vi "Barcode 2D_Main Function.vi"(8 "error in (no error)":errorcluster, 10 "2D Barcode Parameter in":T1={"ROI"={"Global Rectangle"=[], "Contours"=[]}, "Barcode Type"=enum."PDF417", "Data Matrix Parameter"={"Data Matrix Description Options"={"Aspect Ratio"=0.0, "Rows"=0, "Columns"=0, "Rectangle"=FALSE, "ECC"=-2, "Barcode Polarity"=0, "Cell Fill Percentage"=-2, "Minimum Border Integrity %"=80.0, "Mirror Mode"=-2}, "Data Matrix Search Options"={"Rotation Mode"=enum."Unlimited", "Skip Location?"=FALSE, "Edge Threshold"=30, "Demodulation Mode"=-2, "Cell Sample Size"=-2, "Cell Filter Mode"=-2, "Skew Degrees Allowed"=5, "Maximum Iterations"=500, "Initial Search Vector Width"=5}, "Data Matrix Size Options"={"Data Matrix Size"={"Minimum Size"=0, "Maximum Size"=0}, "Quiet Zone Width"=10}, "Advanced Options"=[]}, "PDF147 Search Mode"=enum."Multiple Barcodes", "QR Code Parameter"={"QR Search Options"={"Rotation Mode"=enum."Unlimited", "Skip Location?"=FALSE, "Edge Threshold"=30, "Demodulation Mode"=-2, "Cell Sample Size"=-2, "Cell Filter Mode"=-2, "Skew Degrees Allowed"=5}, "QR Description Options"={"Matrix Size (cells)"=0, "Barcode Polarity"=-2, "Mirror Mode"=-2, "QR Model"=0}, "QR Code Cell Size (pixels)"={"Minimum Size"=3, "Maximum Size"=7}}} {"QR Code Parameter"."QR Description Options"."Mirror Mode" items=["Auto-detect"=-2, "Normal"=0, "Mirrored"=1]; "QR Code Parameter"."QR Description Options"."Matrix Size (cells)" items=["Auto-detect"=0, "11x11 - Version 1 (Micro QR Only)"=11, "13x13 - Version 2 (Micro QR Only)"=13, "15x15 - Version 3 (Micro QR Only)"=15, "17x17 - Version 4 (Micro QR Only)"=17, "21x21 - Version 1"=21, "25x25 - Version 2"=25, "29x29 - Version 3"=29, "33x33 - Version 4"=33, "37x37 - Version 5"=37, "41x41 - Version 6"=41, "45x45 - Version 7"=45, "49x49 - Version 8"=49, "53x53 - Version 9"=53, "57x57 - Version 10"=57, "61x61 - Version 11"=61, "65x65 - Version 12"=65, "69x69 - Version 13"=69, "73x73 - Version 14"=73, "77x77 - Version 15"=77, "81x81 - Version 16"=81, "85x85 - Version 17"=85, "89x89 - Version 18"=89, "93x93 - Version 19"=93, "97x97 - Version 20"=97, "101x101 - Version 21"=101, "105x105 - Version 22"=105, "109x109 - Version 23"=109, "113x113 - Version 24"=113, "117x117 - Version 25"=117, "121x121 - Version 26"=121, "125x125 - Version 27"=125, "129x129 - Version 28"=129, "133x133 - Version 29"=133, "137x137 - Version 30"=137, "141x141 - Version 31"=141, "145x145 - Version 32"=145, "149x149 - Version 33"=149, "153x153 - Version 34"=153, "157x157 - Version 35"=157, "161x161 - Version 36"=161, "165x165 - Version 37"=165, "169x169 -  Version 38"=169, "173x173 - Version 39"=173, "177x177 - Version 40"=177]; "QR Code Parameter"."QR Description Options"."QR Model" items=["Auto-detect", "Micro", "Model 1", "Model 2"]; "QR Code Parameter"."QR Description Options"."Barcode Polarity" items=["Auto-detect"=-2, "Black on White"=0, "White on Black"=1]; "QR Code Parameter"."QR Search Options"."Cell Filter Mode" items=["Auto-detect"=-2, "Average"=0, "Median"=1, "Central Average"=2, "High Average"=3, "Low Average"=4, "Very High Average"=5, "Very Low Average"=6, "All Filters"=8]; "QR Code Parameter"."QR Search Options"."Cell Sample Size" items=["Auto-detect"=-2, "1x1"=1, "2x2"=2, "3x3"=3, "4x4"=4, "5x5"=5, "6x6"=6, "7x7"=7]; "QR Code Parameter"."QR Search Options"."Demodulation Mode" items=["Auto-detect"=-2, "Histogram"=0, "Local Contrast"=1, "Combination"=2, "All"=3]; "Data Matrix Parameter"."Advanced Options"."Value" format="%.2f"; "Data Matrix Parameter"."Data Matrix Search Options"."Cell Filter Mode" items=["Auto-detect"=-2, "Average"=0, "Median"=1, "Central Average"=2, "High Average"=3, "Low Average"=4, "Very High Average"=5, "Very Low Average"=6, "All Filters"=8]; "Data Matrix Parameter"."Data Matrix Search Options"."Cell Sample Size" items=["Auto-detect"=-2, "1x1"=1, "2x2"=2, "3x3"=3, "4x4"=4, "5x5"=5, "6x6"=6, "7x7"=7]; "Data Matrix Parameter"."Data Matrix Search Options"."Demodulation Mode" items=["Auto-detect"=-2, "Histogram"=0, "Local Contrast"=1, "Combination"=2, "All"=3]; "Data Matrix Parameter"."Data Matrix Description Options"."Mirror Mode" items=["Auto-detect"=-2, "Normal"=0, "Mirrored"=1]; "Data Matrix Parameter"."Data Matrix Description Options"."ECC" items=["Auto-detect"=-2, "ECC 000"=0, "ECC 050"=50, "ECC 080"=80, "ECC 100"=100, "ECC 140"=140, "ECC 000-140"=190, "ECC 200"=200]; "Data Matrix Parameter"."Data Matrix Description Options"."Minimum Border Integrity %" format="%.2f"; "Data Matrix Parameter"."Data Matrix Description Options"."Aspect Ratio" format="%.2f"; "Data Matrix Parameter"."Data Matrix Description Options"."Cell Fill Percentage" items=["Auto-detect"=-2, "< 30%"=0, ">= 30%"=1]; "Data Matrix Parameter"."Data Matrix Description Options"."Barcode Polarity" items=["Auto-detect"=-2, "Black on White"=0, "White on Black"=1]}, 11 "Image In":T17) -> (0 "error out":errorcluster, 1 "Bounding Box":cluster{"x":sgl, "y":sgl}[](array[cluster]), 2 "Data":string, 3 "Image Out":T17)   [LabVIEW 2019]
uses:
  <vilib>/vision/Image Controls.llb/IMAQ Image.ctl
  Controls/Barcode 2D/Analysis_Barcode 2D_Parameter.ctl
  <vilib>/vision/Instrument.llb/Data Matrix Description Options.ctl
  <vilib>/vision/Instrument.llb/ECC Type.ctl
  <vilib>/vision/Instrument.llb/Data Matrix Polarity.ctl
  <vilib>/vision/Instrument.llb/Cell Fill Percentage.ctl
  <vilib>/vision/Instrument.llb/Data Matrix Mirror.ctl
  <vilib>/vision/Instrument.llb/Data Matrix Search Options.ctl
  <vilib>/vision/Instrument.llb/Demodulation Mode.ctl
  <vilib>/vision/Instrument.llb/Cell Sample Size.ctl
  <vilib>/vision/Instrument.llb/Cell Filter Mode.ctl
  <vilib>/vision/Instrument.llb/Data Matrix Size Options.ctl
  <vilib>/vision/Instrument.llb/Data Matrix Advanced Options.ctl
  <vilib>/vision/Instrument.llb/QR Code Search Options.ctl
  <vilib>/vision/Instrument.llb/QR Code Description Options.ctl
  <vilib>/vision/Instrument.llb/QR Code Model Type.ctl
  <vilib>/vision/NI_Vision_Development_Module.lvlib
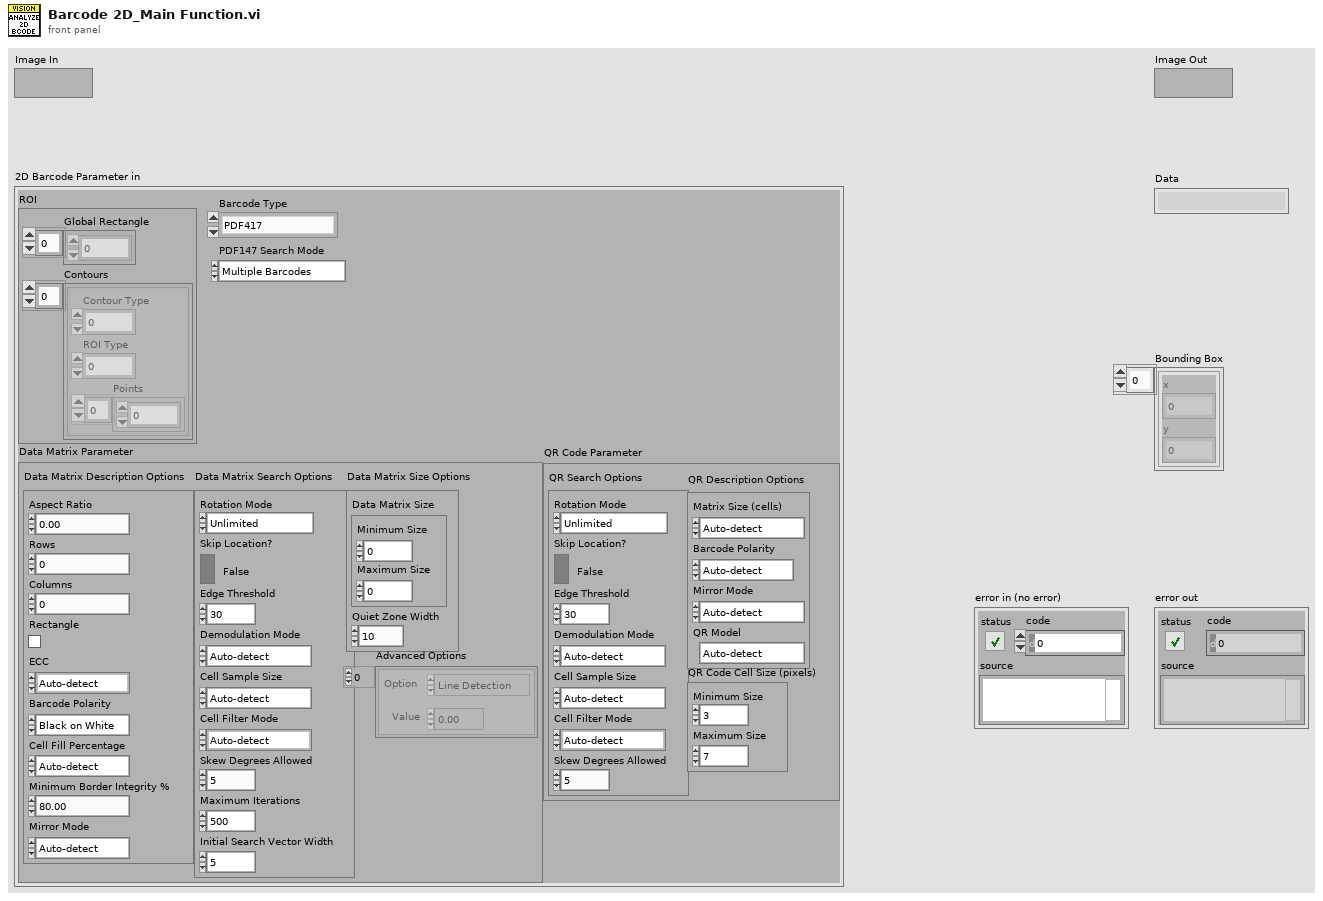
[diagram p1: front panel]
types:
  T1 = typedef "Analysis_Barcode 2D_Parameter.ctl" = cluster{"ROI":cluster{"Global Rectangle":i32[], "Contours":cluster{"Contour Type":u32, "ROI Type":u32, "Points":i32[]}[]}, "Barcode Type":enum16{"Data Matrix", "PDF417", "QR Code"}, "Data Matrix Parameter":cluster{"Data Matrix Description Options":T2, "Data Matrix Search Options":T7, "Data Matrix Size Options":T11, "Advanced Options":T12[]}, "PDF147 Search Mode":T13, "QR Code Parameter":cluster{"QR Search Options":T14, "QR Description Options":T15, "QR Code Cell Size (pixels)":cluster{"Minimum Size":u32, "Maximum Size":u32}}}
  T2 = typedef "Data Matrix Description Options.ctl" = cluster{"Aspect Ratio":sgl, "Rows":u32, "Columns":u32, "Rectangle":bool, "ECC":T3, "Barcode Polarity":T4, "Cell Fill Percentage":T5, "Minimum Border Integrity %":sgl, "Mirror Mode":T6}
  T3 = typedef "ECC Type.ctl" = i32
  T4 = typedef "Data Matrix Polarity.ctl" = i32
  T5 = typedef "Cell Fill Percentage.ctl" = i32
  T6 = typedef "Data Matrix Mirror.ctl" = i32
  T7 = typedef "Data Matrix Search Options.ctl" = cluster{"Rotation Mode":enum32{"Unlimited", "0 Degrees", "90 Degrees", "180 Degrees", "270 Degrees"}, "Skip Location?":bool, "Edge Threshold":u32, "Demodulation Mode":T8, "Cell Sample Size":T9, "Cell Filter Mode":T10, "Skew Degrees Allowed":u32, "Maximum Iterations":u32, "Initial Search Vector Width":u32}
  T8 = typedef "Demodulation Mode.ctl" = i32
  T9 = typedef "Cell Sample Size.ctl" = i32
  T10 = typedef "Cell Filter Mode.ctl" = i32
  T11 = typedef "Data Matrix Size Options.ctl" = cluster{"Data Matrix Size":cluster{"Minimum Size":u32, "Maximum Size":u32}, "Quiet Zone Width":u32}
  T12 = typedef "Data Matrix Advanced Options.ctl" = cluster{"Option":enum32{"Line Detection", "HighLight Filter", "Aggressive", "FNC1", "Refine Bounding Box"}, " Value":dbl}
  T13 = typedef "PDF417 Search Mode" = enum32{"Multiple Barcodes", "Single Barcode, Conservative"}
  T14 = typedef "QR Code Search Options.ctl" = cluster{"Rotation Mode":enum32{"Unlimited", "0 Degrees", "90 Degrees", "180 Degrees", "270 Degrees"}, "Skip Location?":bool, "Edge Threshold":u32, "Demodulation Mode":T8, "Cell Sample Size":T9, "Cell Filter Mode":T10, "Skew Degrees Allowed":u32}
  T15 = typedef "QR Code Description Options.ctl" = cluster{"Matrix Size (cells)":i32, "Barcode Polarity":T4, "Mirror Mode":i32, "QR Model":T16}
  T16 = typedef "QR Code Model Type.ctl" = i32
  T17 = typedef "IMAQ Image.ctl" = refnum<image>
  T18 = cluster{"Global Rectangle":i32[], "Contours":cluster{"Contour Type":u32, "ROI Type":u32, "Points":i32[]}[]}
  T19 = typedef "Data Matrix Report.ctl" = cluster{"Found?":bool, "Binary?":bool, "Data":string, "Bounding Box":cluster{"x":sgl, "y":sgl}[], "Errors Corrected":u32, "Erasures Corrected":u32, "Aspect Ratio":sgl, "Rows":u32, "Columns":u32, "ECC":T3, "Barcode Polarity":T4, "Cell Fill Percentage":T5, "Border Integrity":sgl, "Mirrored?":bool, "Minimum Edge Strength":u32, "Demodulation Mode":T8, "Cell Sample Size":T9, "Cell Filter Mode":T10, "Iterations":u32}
  T20 = typedef "Barcode Report" = cluster{"Type":enum32{"PDF417", "Data Matrix ECC 000", "Data Matrix ECC 050", "Data Matrix ECC 080", "Data Matrix ECC 100", "Data Matrix ECC 140", "Data Matrix ECC 200"}, "Binary":bool, "Data":string, "Bounding Box":cluster{"x":sgl, "y":sgl}[], "Errors Corrected":u32, "Erasures Corrected":u32, "Rows":u32, "Columns":u32}
  T21 = typedef "QR Code Report.ctl" = cluster{"Found?":bool, "Data":string, "Bounding Box":cluster{"x":sgl, "y":sgl}[], "Errors Corrected":u32, "Dimensions (Rows/Cols)":u32, "Version":u32, "QR Model":T16, "Stream Mode":T22, "Barcode Polarity":T4, "Mirrored?":bool, "Append Stream Position":u32, "Size of Append Stream":u32, "First EAN-128 ID":i32, "First Alternate Language ID":i32, "Append Stream ID":u32, "Minimum Edge Strength":u32, "Demodulation Mode":T8, "Cell Sample Size":T9, "Cell Filter Mode":T10}
  T22 = typedef "QR Code Stream Mode Type.ctl" = i32
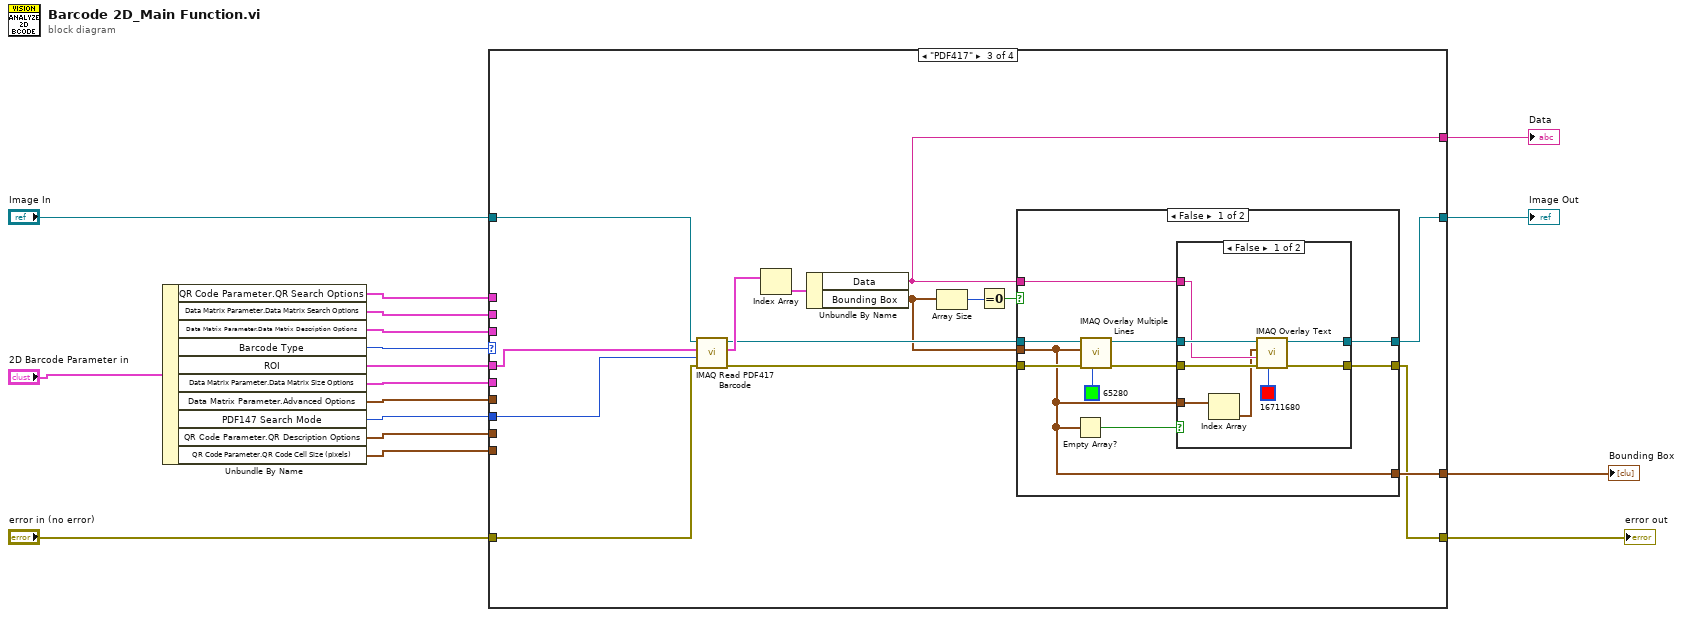
[diagram p0: block diagram]
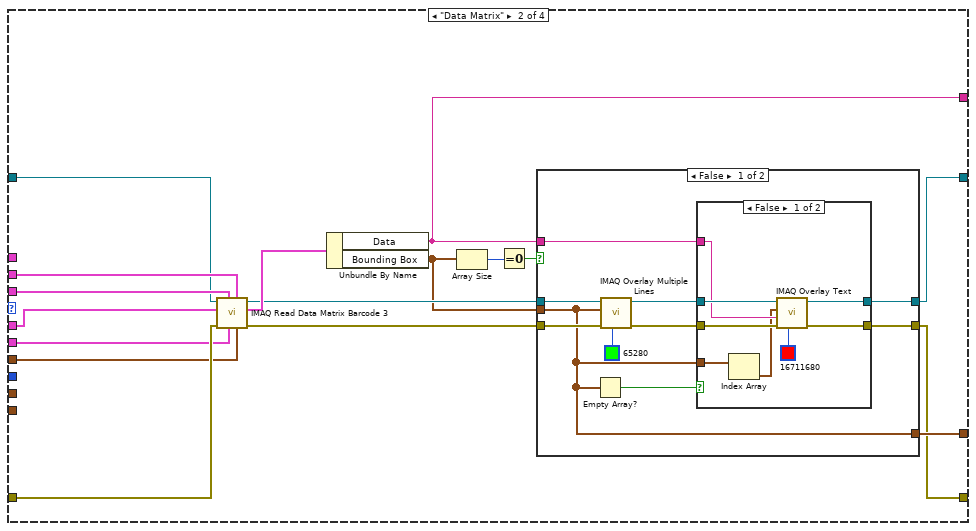
[diagram p3: hidden frame]
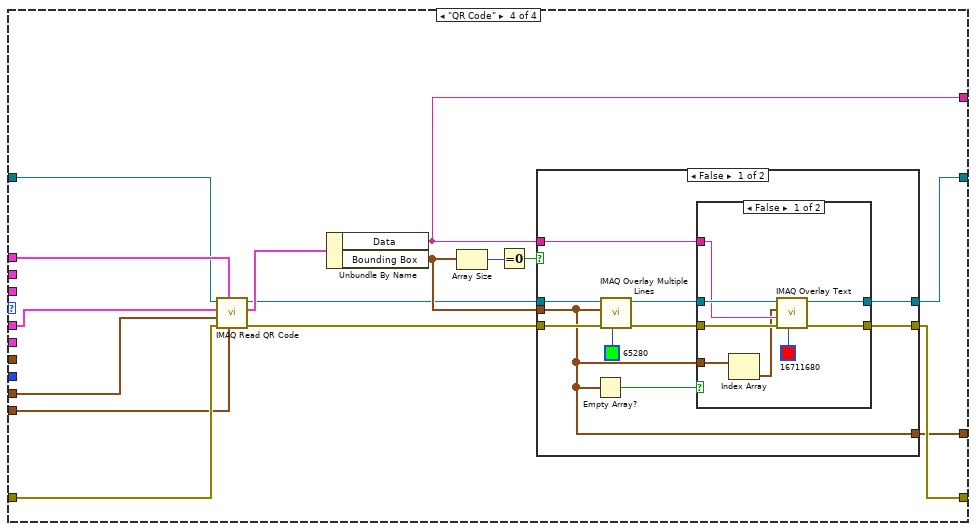
[diagram p8: hidden frame]
diagram:
  n1 = Unbundle By Name("2D Barcode Parameter in") -> ("QR Code Parameter.QR Search Options"=w9:T14, "Data Matrix Parameter.Data Matrix Search Options"=w11:T7, "Data Matrix Parameter.Data Matrix Description Options"=w12:T2, "Barcode Type"=w10:enum16{"Data Matrix", "PDF417", "QR Code"}, "ROI"=w8:T18, "Data Matrix Parameter.Data Matrix Size Options"=w7:T11, "Data Matrix Parameter.Advanced Options"=w6:T12[], "PDF147 Search Mode"=w3:T13, "QR Code Parameter.QR Description Options"=w4:T15, "QR Code Parameter.QR Code Cell Size (pixels)"=w5:cluster{"Minimum Size":u32, "Maximum Size":u32})
  n2 = case shown="\"PDF417\"" w10 {
    tunnel: [w18 w25 w60 w107] -> w1
    tunnel: [w19 w27 w59 w106] -> w17
    tunnel: "error in (no error)" -> [w18 w35 w70 w105]
    tunnel: "Image In" -> [w19 w31 w68 w98]
    tunnel: [_ w26 w61 w102] -> w15
    tunnel: [_ w20 w62 w101] -> w14
    tunnel: w12 -> [_ w33 _ _]
    tunnel: w11 -> [_ w32 _ _]
    tunnel: w9 -> [_ _ _ w100]
    tunnel: w8 -> [_ w30 w69 w99]
    tunnel: w7 -> [_ w29 _ _]
    tunnel: w6 -> [_ w28 _ _]
    tunnel: w4 -> [_ _ _ w96]
    tunnel: w5 -> [_ _ _ w97]
    tunnel: w3 -> [_ _ w67 _]
    frame Default {
    }
    frame "Data Matrix" {
      n3 = call "IMAQ Read Data Matrix Barcode 3"("Advanced Options"=w28, "Data Matrix Search Options"=w32, "Data Matrix Size Options"=w29, "Data Matrix Description Options"=w33, "error in (no error)"=w35, "ROI Descriptor"=w30, "Image"=w31) -> ("error out"=w24:errorcluster, "Data Matrix Report"=w36:T19, "Image (duplicate)"=w23:T17)  [unwired: 1 in, 1 out]
      n4 = Unbundle By Name(w36) -> ("Data"=w20:string, "Bounding Box"=w22:cluster{"x":sgl, "y":sgl}[])
      n5 = Array Size(array=w22) -> (size(s)=w34:i32)
      n6 = Equal To 0?(x=w34) -> (x = 0?=w21:bool)
      n7 = case shown="False" w21 {
        tunnel: w23 -> [w45 w58]
        tunnel: w24 -> [w44 w57]
        tunnel: [w42 w58] -> w27
        tunnel: [w41 w57] -> w25
        tunnel: w22 -> [w38 _]
        tunnel: [w38 _] -> w26
        tunnel: w20 -> [w37 _]
        frame False {
          n8 = Empty Array?(array=w38) -> (empty?=w39:bool)
          n9 = call "IMAQ Overlay Multiple Lines"("Color"=u32 65280, "error in (no error)"=w44, "Line End Points"=w38, "Image"=w45) -> ("error out"=w40:errorcluster, "Image Out"=w43:T17)  [unwired: 6 in]
          n10 = case shown="False" w39 {
            tunnel: w43 -> [w54 w55]
            tunnel: [w53 w55] -> w42
            tunnel: [w52 w56] -> w41
            tunnel: w40 -> [w51 w56]
            tunnel: w38 -> [w48 _]
            tunnel: w37 -> [w50 _]
            frame False {
              n11 = Index Array(array=w48) -> (element=w47:cluster{"x":sgl, "y":sgl})  [unwired: 1 in]
              n12 = call "IMAQ Overlay Text"("Text Color (black)"=u32 16711680, "error in (no error)"=w51, "String"=w50, "Origin"=w47, "Image"=w54) -> ("error out"=w52:errorcluster, "Image Out"=w53:T17)  [unwired: 5 in]
            }
            frame True {
            }
          }
        }
        frame True {
        }
      }
    }
    frame "PDF417" {
      n13 = call "IMAQ Read PDF417 Barcode"("error in (no error)"=w70, "Search Mode"=w67, "ROI Descriptor"=w69, "Image"=w68) -> ("error out"=w64:errorcluster, "Barcodes"=w73:T20[], "Image (duplicate)"=w65:T17)  [unwired: 4 in, 1 out]
      n14 = Index Array(array=w73) -> (element=w72:T20)  [unwired: 1 in]
      n15 = Unbundle By Name(w72) -> ("Data"=w62:string, "Bounding Box"=w63:cluster{"x":sgl, "y":sgl}[])
      n16 = Array Size(array=w63) -> (size(s)=w71:i32)
      n17 = Equal To 0?(x=w71) -> (x = 0?=w66:bool)
      n18 = case shown="False" w66 {
        tunnel: w65 -> [w82 w95]
        tunnel: w64 -> [w81 w94]
        tunnel: [w79 w95] -> w59
        tunnel: [w78 w94] -> w60
        tunnel: w63 -> [w75 _]
        tunnel: [w75 _] -> w61
        tunnel: w62 -> [w74 _]
        frame False {
          n19 = Empty Array?(array=w75) -> (empty?=w76:bool)
          n20 = call "IMAQ Overlay Multiple Lines"("Color"=u32 65280, "error in (no error)"=w81, "Line End Points"=w75, "Image"=w82) -> ("error out"=w77:errorcluster, "Image Out"=w80:T17)  [unwired: 6 in]
          n21 = case shown="False" w76 {
            tunnel: w80 -> [w91 w92]
            tunnel: [w90 w92] -> w79
            tunnel: [w89 w93] -> w78
            tunnel: w77 -> [w88 w93]
            tunnel: w75 -> [w85 _]
            tunnel: w74 -> [w87 _]
            frame False {
              n22 = Index Array(array=w85) -> (element=w84:cluster{"x":sgl, "y":sgl})  [unwired: 1 in]
              n23 = call "IMAQ Overlay Text"("Text Color (black)"=u32 16711680, "error in (no error)"=w88, "String"=w87, "Origin"=w84, "Image"=w91) -> ("error out"=w89:errorcluster, "Image Out"=w90:T17)  [unwired: 5 in]
            }
            frame True {
            }
          }
        }
        frame True {
        }
      }
    }
    frame "QR Code" {
      n24 = call "IMAQ Read QR Code"("QR Code Cell Size (pixels)"=w97, "QR Search Options"=w100, "error in (no error)"=w105, "QR Description Options"=w96, "ROI Descriptor"=w99, "Image"=w98) -> ("error out"=w104:errorcluster, "QR Code Report"=w108:T21, "Image (duplicate)"=w103:T17)  [unwired: 2 in, 1 out]
      n25 = Unbundle By Name(w108) -> ("Data"=w101:string, "Bounding Box"=w111:cluster{"x":sgl, "y":sgl}[])
      n26 = Array Size(array=w111) -> (size(s)=w109:i32)
      n27 = Equal To 0?(x=w109) -> (x = 0?=w110:bool)
      n28 = case shown="False" w110 {
        tunnel: w103 -> [w120 w133]
        tunnel: w104 -> [w119 w132]
        tunnel: [w117 w133] -> w106
        tunnel: [w116 w132] -> w107
        tunnel: w111 -> [w113 _]
        tunnel: [w113 _] -> w102
        tunnel: w101 -> [w112 _]
        frame False {
          n29 = Empty Array?(array=w113) -> (empty?=w114:bool)
          n30 = call "IMAQ Overlay Multiple Lines"("Color"=u32 65280, "error in (no error)"=w119, "Line End Points"=w113, "Image"=w120) -> ("error out"=w115:errorcluster, "Image Out"=w118:T17)  [unwired: 6 in]
          n31 = case shown="False" w114 {
            tunnel: w118 -> [w129 w130]
            tunnel: [w128 w130] -> w117
            tunnel: [w127 w131] -> w116
            tunnel: w115 -> [w126 w131]
            tunnel: w113 -> [w123 _]
            tunnel: w112 -> [w125 _]
            frame False {
              n32 = Index Array(array=w123) -> (element=w122:cluster{"x":sgl, "y":sgl})  [unwired: 1 in]
              n33 = call "IMAQ Overlay Text"("Text Color (black)"=u32 16711680, "error in (no error)"=w126, "String"=w125, "Origin"=w122, "Image"=w129) -> ("error out"=w127:errorcluster, "Image Out"=w128:T17)  [unwired: 5 in]
            }
            frame True {
            }
          }
        }
        frame True {
        }
      }
    }
  }
  "Image Out" <- w17
  "Bounding Box" <- w15
  "Data" <- w14
  "error out" <- w1
